vi "solar DeQ.vi"(8 "error in (no error)":errorcluster, 9 "ms Timeout (-1)":i32=-1, 10 "Timeout CMD (\"\")":cluster{"MSG":string, "DATA":variant}, 11 "solar in":refnum<class "solar.lvclass">) -> (0 "error out":errorcluster, 1 "DATA":variant, 2 "MSG":string, 3 "solar out":refnum<class "solar.lvclass">, 5 "Timed Out?":bool)   [LabVIEW 2018, in "solar.lvclass"]
doc: "This dequeues the next target message. Use the optional override VIs to unpack and handle interlock checks before the command is returned. If the command is send locally (i.e. No 'HDR_GUID' attribute), this relays the message to COSMOS. Lastly, all commands get recorded in the SOLAR log."
uses:
  solar.lvclass
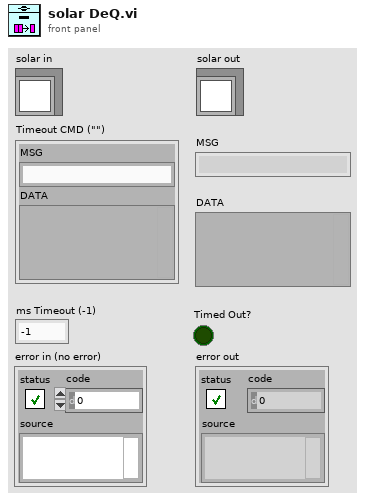
[diagram p1: front panel]
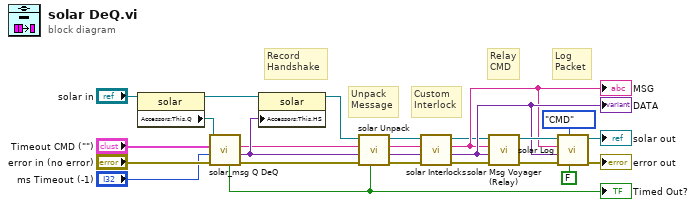
[diagram p0: block diagram]
diagram:
  # "Custom\nInterlock"
  # "Record\nHandshake"
  # "Log\nPacket"
  # "Unpack\nMessage"
  # "Relay\nCMD"
  n1 = property class="solar"(reference="solar in") -> (reference out=w19:refnum<class "solar.lvclass">, "Accessors:This.Q"=w18:refnum<queue>)  [unwired: 1 in, 1 out]
  n2 = call "solar_msg Q DeQ.vi"("error in (no error)"="error in (no error)", "Timeout ms (-1)"="ms Timeout (-1)", "CMD Timeout (\"\")"="Timeout CMD (\"\")", "Queue in"=w18) -> ("error out"=w8:errorcluster, "CMD_DATA"=w7:variant, "CMD"=w6:string, "Timed Out?"=w1:bool)  [unwired: 3 in, 1 out]
  "Timed Out?" <- w1
  n3 = property class="solar"(reference=w19, "Accessors:This.HS"=w7) -> (reference out=w9:refnum<class "solar.lvclass">)  [unwired: 1 in, 1 out]
  n4 = call-dynamic "solar Unpack.vi"("Timed Out?"=w1, "error in (no error)"=w8, "DATA in"=w7, "MSG in"=w6, "solar in"=w9) -> ("error out"=w10:errorcluster, "DATA out"=w11:variant, "MSG out"=w12:string, "solar out"=w13:refnum<class "solar.lvclass">)  [unwired: 3 in]
  n5 = call-dynamic "solar Interlocks.vi"("error in (no error)"=w10, "DATA in"=w11, "MSG in"=w12, "solar in"=w13) -> ("error out"=w5:errorcluster, "DATA out"=w4:variant, "MSG out"=w3:string, "solar out"=w2:refnum<class "solar.lvclass">)  [unwired: 4 in]
  "MSG" <- w3
  "DATA" <- w4
  n6 = call "solar Msg Voyager (Relay).vi"("error in (no error)"=w5, "CMD_DATA"=w4, "CMD"=w3, "solar in"=w2) -> ("error out"=w17:errorcluster, "solar out"=w16:refnum<class "solar.lvclass">)  [unwired: 6 in]
  n7 = call "solar Log.vi"("Clear Error? (T)"=FALSE ("Clear Error?"), "Type (TLM)"=enum8{"CMD", "TLM"}."CMD" ("Type (CMD)"), "error in (no error)"=w17, "DATA"=w4, "MSG"=w3, "solar in"=w16) -> ("error out"=→"error out":errorcluster, "solar out"=→"solar out":refnum<class "solar.lvclass">)  [unwired: 4 in]
